vi "GetChannelBandwidth.vi"(8 "error in (no error)":errorcluster, 11 "TektronixDPO_PhysicalDevice.lvclass":refnum<class "TektronixDPO_PhysicalDevice.lvclass">) -> (0 "error out":errorcluster, 3 "TektronixDPO_PhysicalDevice.lvclassOut":refnum<class "TektronixDPO_PhysicalDevice.lvclass">)   [LabVIEW 2013, in "TektronixDPO_PhysicalDevice.lvclass"]
doc: "Read from the phsyical device the offset relative to the specified channel"
uses:
  TektronixDPO_PhysicalDevice.lvclass
  shared/Typdefs/Choice79.ctl
  TektronixDPO_PhysicalDevice.lvclass/TektronixDPO_PhysicalDevice.ctl
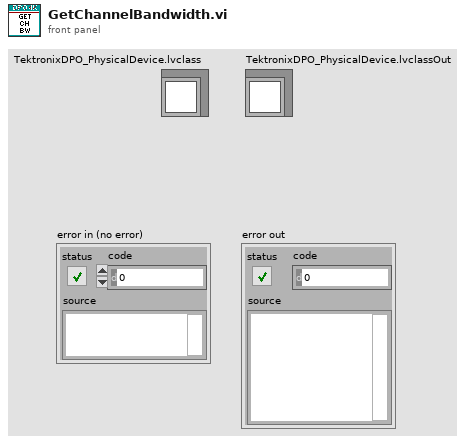
[diagram p1: front panel]
types:
  T1 = typedef "Choice79.ctl" = enum16{"FULL", "250 MHz", "150 MHz", "20 MHz"}
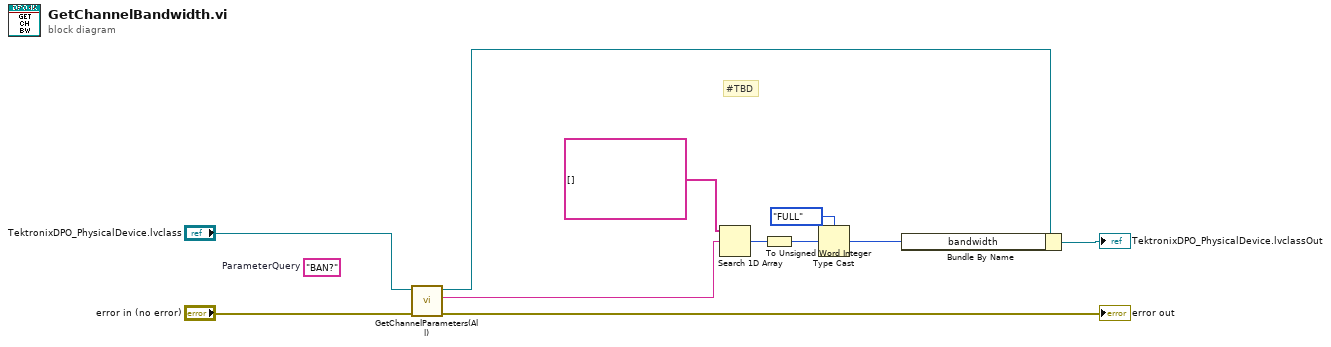
[diagram p0: block diagram]
diagram:
  (unwired) "BAN?"  # ParameterQuery
  # "#TBD"
  n1 = call "GetChannelParameters(All).vi"("error in (no error)"="error in (no error)", "TektronixDPO_PhysicalDevice in"="TektronixDPO_PhysicalDevice.lvclass") -> ("error out"=→"error out":errorcluster, "Response"=w8:string, "TektronixDPO_PhysicalDevice out"=w1:refnum<class "TektronixDPO_PhysicalDevice.lvclass">)  [unwired: 7 in]
  n2 = Search 1D Array(1D array=string[] [], element=w8) -> (index of element=w7:i32)  [unwired: 1 in]
  n3 = To Unsigned Word Integer(number=w7) -> (unsigned 16bit integer=w6:u16)
  n4 = Type Cast(type=Choice79."FULL" ("Channel0"), x=w6) -> (*(type *) &x=w3:T1)
  n5 = Bundle By Name(cluster=w1, "bandwidth"=w3) -> (→"TektronixDPO_PhysicalDevice.lvclassOut":refnum<class "TektronixDPO_PhysicalDevice.lvclass">)
